vi "Spawn Logic.vi"(7 "Actor in":refnum<class "Actor.lvclass">, 10 "Spawn Logic":T1={"Actor Layers"=[], "UID"="", "Transport"=refnum, "Root"=FALSE, "Stop When Parent Stopped"=TRUE}) -> (0 "Error out":errorcluster, 5 "Actor out":refnum<class "Actor.lvclass">)   [LabVIEW 2025, in "jettl.lvlib"]
uses:
  jettl.lvlib
  Actor/Actor.lvclass
  Spawn Logic.ctl
  Transport/Transport/Transport.lvclass
  Core Actor/Core Actor.lvlib
  Error/Error.lvlib
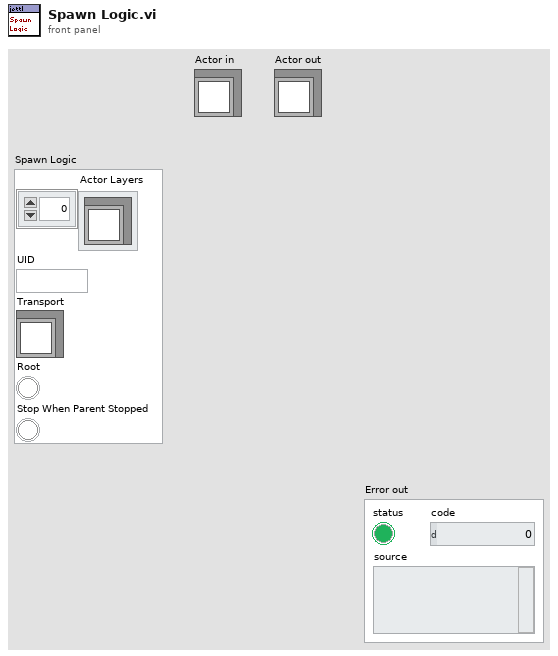
[diagram p1: front panel]
types:
  T1 = typedef "jettl.lvlib/Spawn Logic.ctl" = cluster{"Actor Layers":refnum<class "Actor.lvclass">[], "UID":string, "Transport":refnum<class "Transport.lvclass">, "Root":bool, "Stop When Parent Stopped":bool}
  T2 = typedef "jettl.lvlib/Child UIDs.ctl" = set{string}
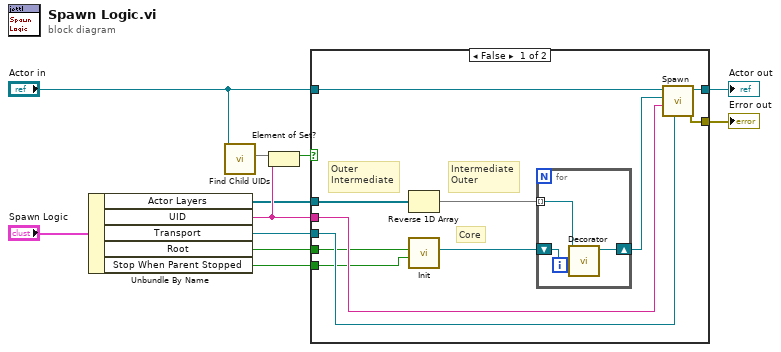
[diagram p0: block diagram]
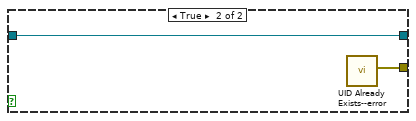
[diagram p2: hidden frame]
diagram:
  n1 = Unbundle By Name("Spawn Logic") -> ("Actor Layers"=w4:refnum<class "Actor.lvclass">[], "UID"=w5:string, "Transport"=w6:refnum<class "Transport.lvclass">, "Root"=w2:bool, "Stop When Parent Stopped"=w3:bool)
  n2 = call-dynamic "Find Child UIDs.vi"("Actor in"="Actor in") -> ("Child UIDs"=w11:T2)  [unwired: 10 in]
  n3 = Element of Set?(10:w5, 11:w11) -> (3:w1:bool)
  n4 = case shown="False" w1 {
    tunnel: w5 -> [w19 _]
    tunnel: "Actor in" -> [w20 w27]
    tunnel: [w22 w26] -> w9
    tunnel: [w21 w27] -> w10
    tunnel: w6 -> [w18 _]
    tunnel: w4 -> [w15 _]
    tunnel: w3 -> [w14 _]
    tunnel: w2 -> [w13 _]
    frame False {
      # "Intermediate\nOuter"
      # "Outer\nIntermediate"
      # "Core"
      n5 = Reverse 1D Array(array=w15) -> (reversed array=w16:refnum<class "Actor.lvclass">[])
      n6 = call "Init.vi"("Stop When Parent Stopped"=w14, "Root"=w13) -> ("Actor"=w17:refnum<class "Actor.lvclass">)  [unwired: 9 in]
      n7 = for {
        tunnel: w16 -> [w24] mode=indexing
        shift-right: [w23] -> w12
        shift-left: w17 -> [w25]
        n8 = call-dynamic "Decorator.vi"("Actor"=w25, "Actor in"=w24) -> ("Actor out"=w23:refnum<class "Actor.lvclass">)  [unwired: 9 in]
      }
      n9 = call-dynamic "Spawn.vi"("Transport"=w18, "UID"=w19, "Actor"=w12, "Actor in"=w20) -> ("Error out"=w22:errorcluster, "Actor out"=w21:refnum<class "Actor.lvclass">)  [unwired: 6 in]
    }
    frame True {
      n10 = call "UID Already Exists--error.vi"() -> ("Error"=w26:errorcluster)  [unwired: 11 in]
    }
  }
  "Actor out" <- w10
  "Error out" <- w9
